vi "GSI-HVSwitch2.emergency off.vi"(0 "i ref in":refnum<vi>, 3 "ms timeout (10000)":i32=10000, 5 "error in (no error)":errorcluster) -> (14 "i ref out":refnum<vi>, 17 "timed out":bool, 19 "error out":errorcluster)   [LabVIEW 2014, in "GSI-HVSwitch2.lvlib"]
doc: "Performs an emergency OFF by setting the voltages to 0 and by switching off amplifier of the power supply."
uses:
  GSI-HVSwitch2.lvlib
  CS_Core/CSApplicationBaseClasses/DeviceBase/DeviceBase.lvlib
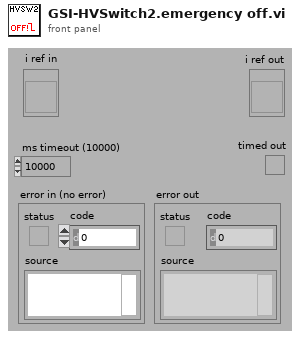
[diagram p1: front panel]
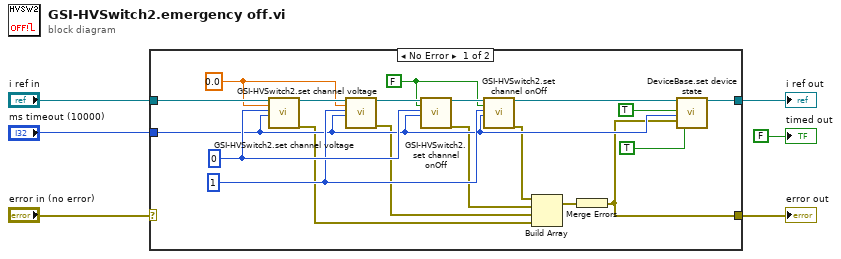
[diagram p0: block diagram]
diagram:
  n1 = case shown="No Error" "error in (no error)" {
    selector: "error in (no error)" -> [_ w26]
    tunnel: "i ref in" -> [w25 w27]
    tunnel: [w22 w27] -> w5
    tunnel: "ms timeout (10000)" -> [w14 _]
    tunnel: [w13 w26] -> w2
    frame No Error {
      w23 = 0.0 ("nomVoltage")
      w15 = FALSE ("on (FALSE)")
      w16 = 1 ("channel")
      w18 = 0 ("channel")
      n2 = call "GSI-HVSwitch2.set channel voltage.vi"("i ref in"=w25, "nomVoltage"=w23, "channel"=w18, "ms timeout (10000)"=w14) -> ("i ref out"=w24:refnum<vi>, "error out"=w9:errorcluster)  [unwired: 13 in, 1 out]
      n3 = call "GSI-HVSwitch2.set channel voltage.vi"("i ref in"=w24, "nomVoltage"=w23, "channel"=w16, "ms timeout (10000)"=w14) -> ("i ref out"=w19:refnum<vi>, "error out"=w10:errorcluster)  [unwired: 13 in, 1 out]
      n4 = call "GSI-HVSwitch2.set channel onOff.vi"("i ref in"=w19, "on (FALSE)"=w15, "channel"=w18, "ms timeout (10000)"=w14) -> ("i ref out"=w17:refnum<vi>, "error out"=w11:errorcluster)  [unwired: 13 in, 1 out]
      n5 = call "GSI-HVSwitch2.set channel onOff.vi"("i ref in"=w17, "on (FALSE)"=w15, "channel"=w16, "ms timeout (10000)"=w14) -> ("i ref out"=w7:refnum<vi>, "error out"=w12:errorcluster)  [unwired: 13 in, 1 out]
      n6 = Build Array(w12, w11, w10, w9) -> (w8:errorcluster[])
      n7 = Merge Errors(w8) -> (w13:errorcluster)
      n8 = call "DeviceBase.set device state.vi"("i ref in"=w7, "implicit"=TRUE, "ms timeout (10000)"=w14, "device error"=w13, "mayResetError (FALSE)"=TRUE) -> ("i ref out"=w22:refnum<vi>)  [unwired: 12 in, 2 out]
    }
    frame Error {
    }
  }
  "error out" <- w2
  "i ref out" <- w5
  "timed out" <- FALSE ("timed out")
